vi "GHV232 CRAB Send Data.vi"(1 "Reset":bool, 2 "Send":bool, 4 "Version":bool, 5 "HV Enable":bool, 6 "Current Program":dbl min=0.0 max=100.0 step=0.1 format="%#.2g", 7 "Voltage Program":dbl min=0.0 max=100.0 step=0.1 format="%#.2g", 8 "error in (no error)":errorcluster, 11 "VISA resource name":refnum<visa-resource-name>) -> (0 "error out":errorcluster, 3 "VISA resource name 2":refnum<visa-resource-name>)   [LabVIEW 2017]
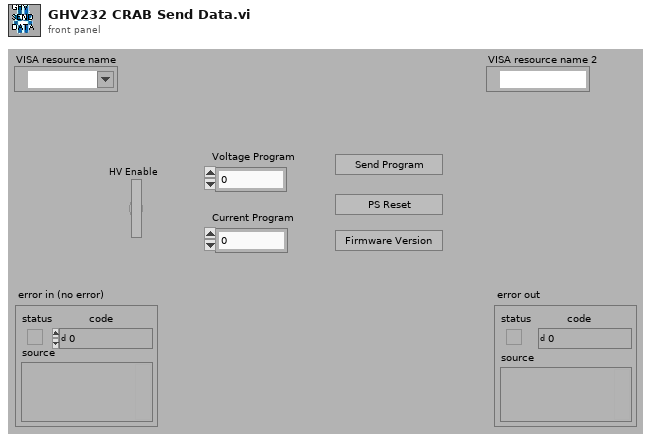
[diagram p1: front panel]
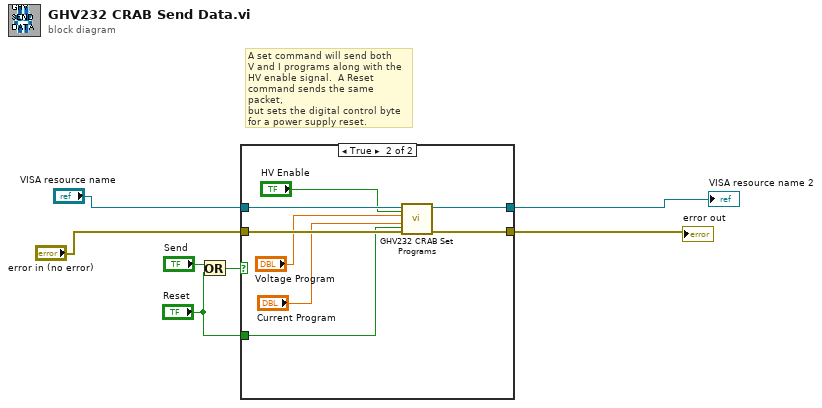
[diagram p0: block diagram]
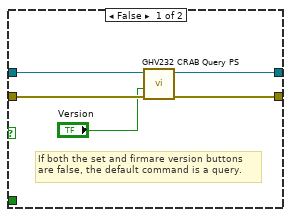
[diagram p2: hidden frame]
diagram:
  # "A set command will send both\nV and I programs along with the\nHV enable signal.  A Reset \ncommand sends the same packet,\nbut sets the digital control byte\nfor a power supply reset."
  n1 = Or(x="Send", y="Reset") -> (x .or. y?=w7:bool)
  n2 = case shown="True" w7 {
    tunnel: [w9 w18] -> w3
    tunnel: "VISA resource name" -> [w12 w20]
    tunnel: "error in (no error)" -> [w11 w19]
    tunnel: [w10 w17] -> w4
    tunnel: "Reset" -> [_ w16]
    frame False {
      # "If both the set and firmare version buttons\nare false, the default command is a query."
      n3 = call "GHV232 CRAB Query PS.vi"("error in (no error)"=w11, "Version"="Version", "VISA resource name"=w12) -> ("error out"=w9:errorcluster, "VISA resource name 2"=w10:refnum<visa-resource-name>)  [unwired: 7 in]
    }
    frame True {
      n4 = call "GHV232 CRAB Set Programs.vi"(6:w16, "HV on"="HV Enable", "error in (no error)"=w19, "I prog"="Current Program", "V prog"="Voltage Program", "VISA resource name"=w20) -> ("error out"=w18:errorcluster, "VISA resource name 2"=w17:refnum<visa-resource-name>)  [unwired: 4 in]
    }
  }
  "VISA resource name 2" <- w4
  "error out" <- w3
